vi "laser_only.vi"() -> ()   [LabVIEW 2010]
panel:
  out "Status":string
  in  "ITI duration (sec)":dbl=25.0
  in  "laser duration (sec)":dbl=5.0
  in  "laser port":tag="Dev1/port1/line6"
  in  "stand-by duration (sec)":dbl=30.0
  in  "stop":bool
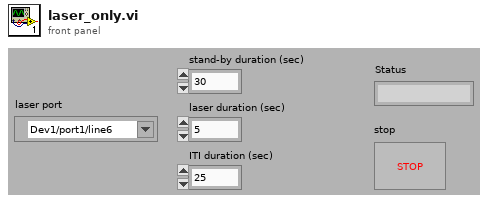
[diagram p1: front panel]
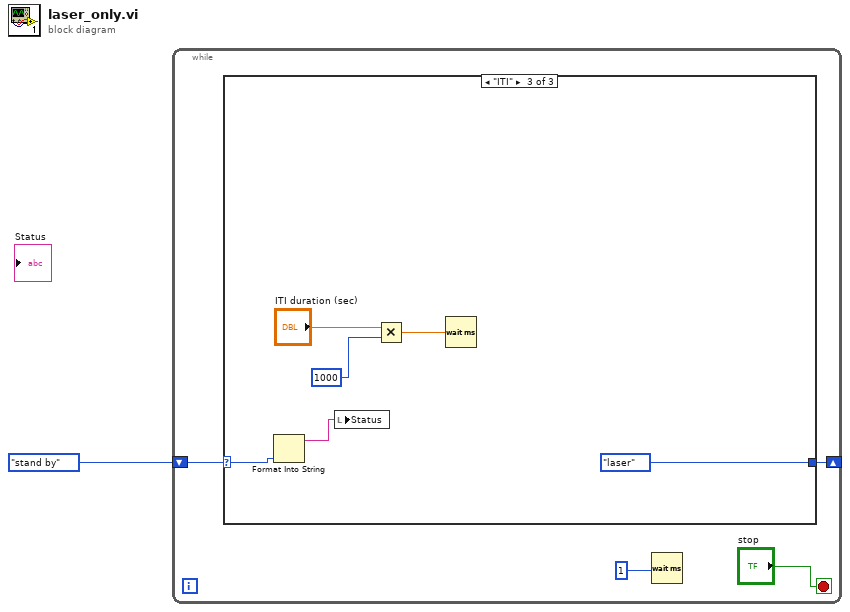
[diagram p0: block diagram]
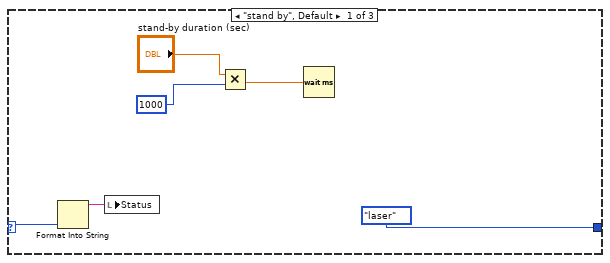
[diagram p2: hidden frame]
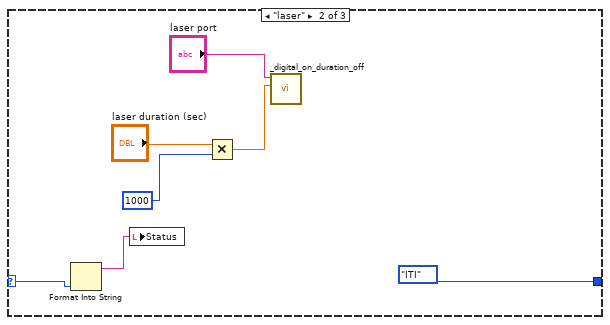
[diagram p3: hidden frame]
diagram:
  n1 = while {
    shift-right: [w3] -> _
    shift-left: enum16{"stand by", "laser", "ITI"}."stand by" -> [w4]
    stop <- "stop" stop-if-true
    n2 = case shown="\"ITI\"" w4 {
      selector: w4 -> [w6 w12 w19]
      tunnel: [enum16{"stand by", "laser", "ITI"}."laser" enum16{"stand by", "laser", "ITI"}."ITI" enum16{"stand by", "laser", "ITI"}."laser"] -> w3
      frame "stand by", Default {
        n3 = Format Into String(w6) -> (resulting string=w7:string)  [unwired: 3 in, 1 out]
        n4 = local write "Status"(w7) -> ()
        n5 = Multiply(x="stand-by duration (sec)", y=1000) -> (x*y=w11:dbl)
        n6 = Wait (ms)(milliseconds to wait=w11) -> ()  [unwired: 1 out]
      }
      frame "laser" {
        n7 = Format Into String(w12) -> (resulting string=w13:string)  [unwired: 3 in, 1 out]
        n8 = local write "Status"(w13) -> ()
        n9 = Multiply(x="laser duration (sec)", y=1000) -> (x*y=w15:dbl)
        n10 = call "_digital_on_duration_off.vi"("duration (ms)"=w15, "digital port"="laser port") -> ()  [unwired: 10 in]
      }
      frame "ITI" {
        n11 = Format Into String(w19) -> (resulting string=w20:string)  [unwired: 3 in, 1 out]
        n12 = local write "Status"(w20) -> ()
        n13 = Multiply(x="ITI duration (sec)", y=1000) -> (x*y=w22:dbl)
        n14 = Wait (ms)(milliseconds to wait=w22) -> ()  [unwired: 1 out]
      }
    }
    n15 = Wait (ms)(milliseconds to wait=1) -> ()  [unwired: 1 out]
  }
